vi "Load XCL template.vi"(9 "Template definition":T1={"Keywords column"=0, "Sig. freq. column"=1, "Rec. len. column"=2, "Meas. points. row min to read"=9, "Meas. points. row max to read"=1509, "Properties column"=4, "Properties row start"=1, "Properties row end"=5, "Keyword START regexp"="[Ss][Tt][Aa][Rr][Tt]", "Keyword STOP regexp"="[Ss][Tt][Oo][Pp]"}, 10 "Measurement template file":path, 11 "Measurement properties":T2={"Measurement frequencies (Hz)"=[1000.0, 10000.0, 1000.0], "Sampling frequency (Hz)"=500000.0, "Signal amplitude (V)"=4.5, "AC-DC settle time (s)"=20.0, "Record length (multiples of period)"=[1000.0, 10000.0, 1000.0], "Measurement template file"=path "", "Row of START keyword"=0, "Row of STOP keyword"=0, "Calculate RMS from samples"=FALSE, "AC-DC warm up time (s)"=300.0, "Measurement template line"=[], "DC meter readings No."=10} {"Record length (multiples of period)" format="%#_3p"; "Sampling frequency (Hz)" format="%#_3p"; "Measurement frequencies (Hz)" format="%#_3p"}) -> (3 "Measurement properties out":T2={"Measurement frequencies (Hz)"=[1000.0, 10000.0, 1000.0], "Sampling frequency (Hz)"=500000.0, "Signal amplitude (V)"=4.5, "AC-DC settle time (s)"=20.0, "Record length (multiples of period)"=[1000.0, 10000.0, 1000.0], "Measurement template file"=path "", "Row of START keyword"=0, "Row of STOP keyword"=0, "Calculate RMS from samples"=FALSE, "AC-DC warm up time (s)"=300.0, "Measurement template line"=[], "DC meter readings No."=10} {"Record length (multiples of period)" format="%#_3p"; "Sampling frequency (Hz)" format="%#_3p"; "Measurement frequencies (Hz)" format="%#_3p"})   [LabVIEW 2020]
doc: "Reads values from measurement template in excell spreadsheet."
uses:
  Measurement/Type definitions/Measuement properties.ctl
  Type definitions/Template definition.ctl
  <vilib>/Utility/NIReport.llb/Report Type.ctl
  <vilib>/Utility/error.llb/DialogType.ctl
  <vilib>/addons/_office/excel.llb/Excel Get Data ([str]).vi
  <vilib>/Utility/NIReport.llb/NI_report.lvclass
  <vilib>/addons/_office/NI_ReportGenerationToolkit.lvlib
  <vilib>/Utility/NIReport.llb/NI_ReportGenerationCore.lvlib
  <vilib>/Utility/NIReport.llb/Excel/NI_Excel.lvclass
panel:
  out "Stop row":i32
  out "Start row":i32
  out "excell template content":string[][](array[string])
  out "error out":errorcluster
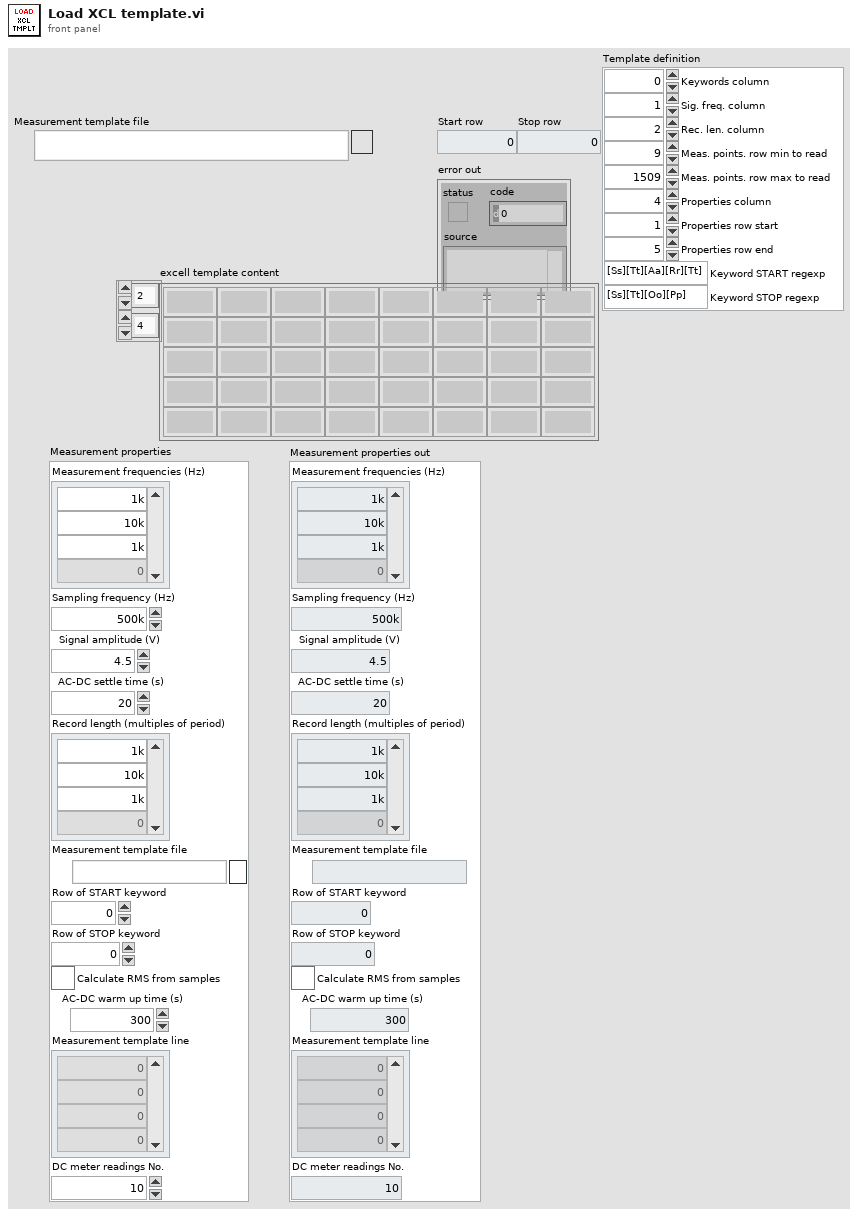
[diagram p1: front panel]
types:
  T1 = typedef "Template definition.ctl" = cluster{"Keywords column":i32, "Sig. freq. column":i32, "Rec. len. column":i32, "Meas. points. row min to read":i32, "Meas. points. row max to read":i32, "Properties column":i32, "Properties row start":i32, "Properties row end":i32, "Keyword START regexp":string, "Keyword STOP regexp":string}
  T2 = typedef "Measuement properties.ctl" = cluster{"Measurement frequencies (Hz)":dbl[], "Sampling frequency (Hz)":dbl, "Signal amplitude (V)":dbl, "AC-DC settle time (s)":dbl, "Record length (multiples of period)":dbl[], "Measurement template file":path, "Row of START keyword":i32, "Row of STOP keyword":i32, "Calculate RMS from samples":bool, "AC-DC warm up time (s)":dbl, "Measurement template line":i32[], "DC meter readings No.":i32}
  T3 = enum16{"maximized", "minimized", "normal", "no change"}
  T4 = typedef "NI_ReportGenerationCore.lvlib/Report Type.ctl" = enum16{"HTML", "Word", "Excel"}
  T5 = typedef "DialogType.ctl" = u16
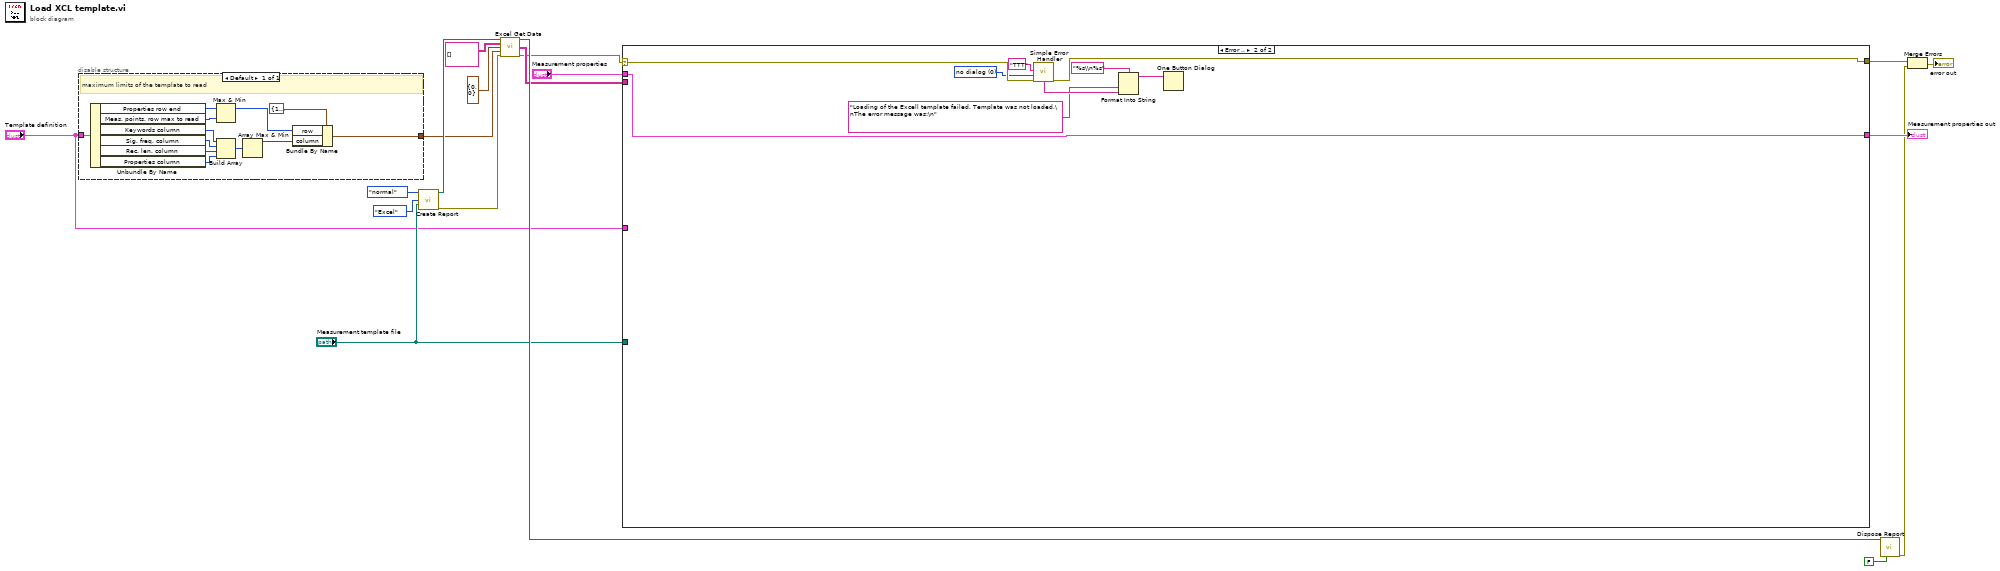
[diagram p0: block diagram]
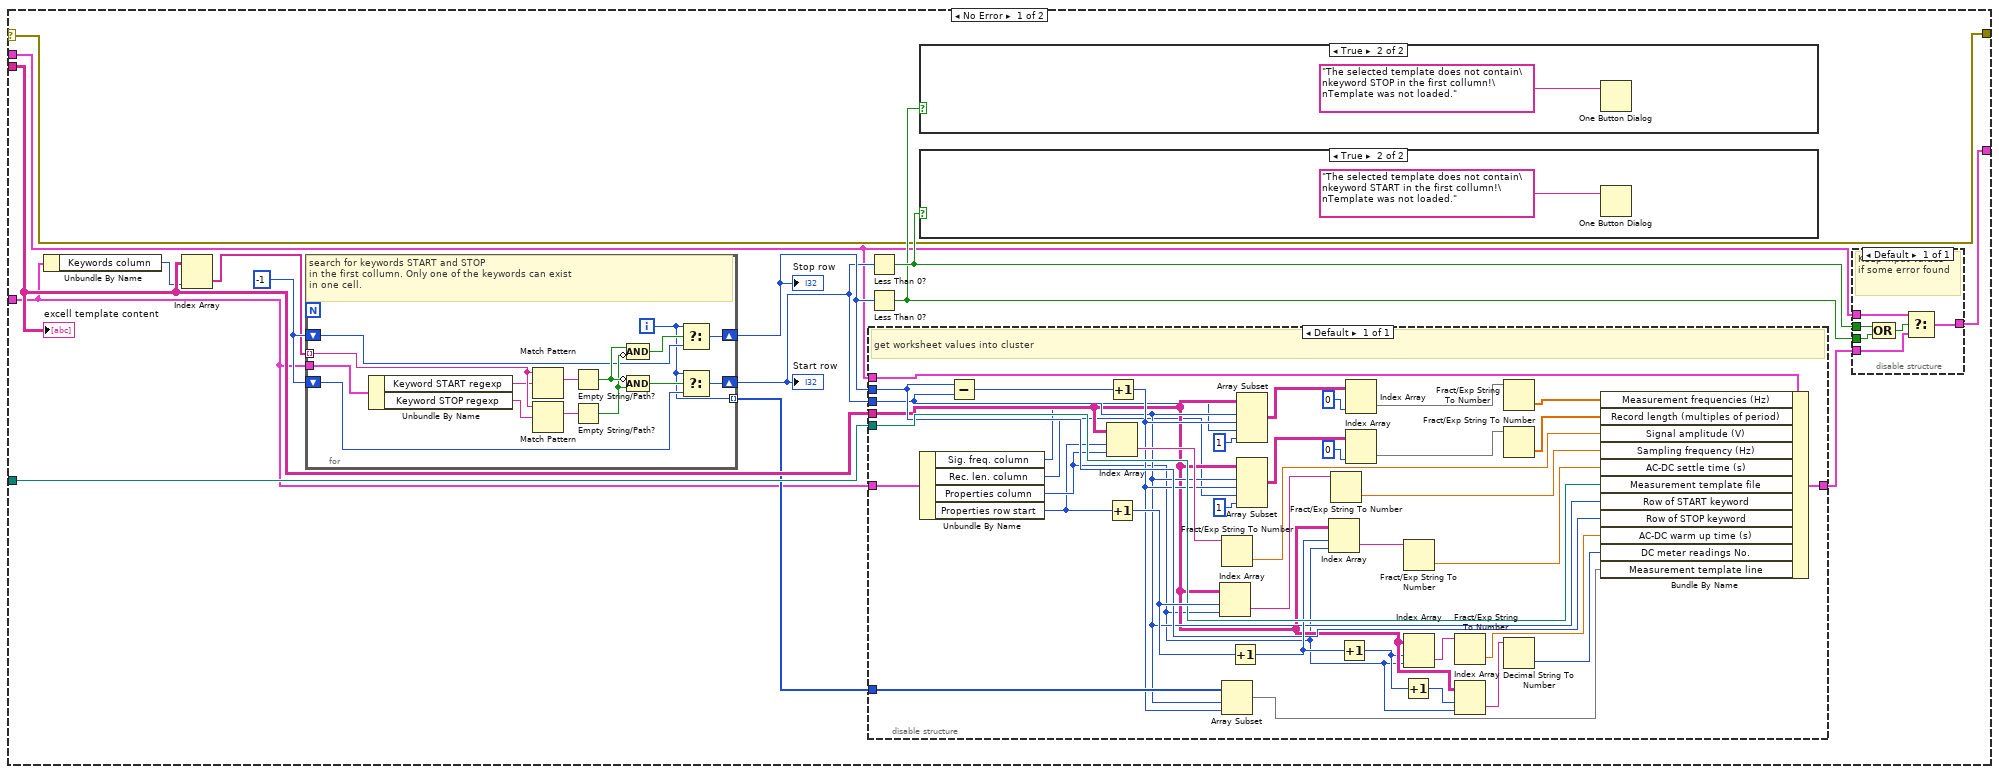
[diagram p2: hidden frame]
diagram:
  n1 = disable-structure shown="Default" {
    disable-tunnel: "Template definition" -> [w30]
    disable-tunnel: [w28] -> w2
    frame Enabled {
      # "maximum limits of the template to read"
      n2 = Unbundle By Name(w30) -> ("Properties row end"=w21:i32, "Meas. points. row max to read"=w20:i32, "Keywords column"=w27:i32, "Sig. freq. column"=w26:i32, "Rec. len. column"=w25:i32, "Properties column"=w24:i32)
      n3 = Max & Min(x=w21, y=w20) -> (max(x,y)=w19:i32)  [unwired: 1 out]
      n4 = Build Array(w27, w26, w25, w24) -> (w23:i32[])
      n5 = Array Max & Min(array=w23) -> (max value=w22:i32)  [unwired: 3 out]
      n6 = Bundle By Name(cluster=cluster{"row":i32, "column":i32} {"row"=100000, "column"=7} ("end (-1, -1)"), "row"=w19, "column"=w22) -> (w28:cluster{"row":i32, "column":i32})
    }
  }
  n7 = call <vilib>:"Create Report.vi"("window state (normal)"=T3."normal", "report type"=Report_Type."Excel", "template (empty)"="Measurement template file") -> ("report out"=w18:refnum<class "NI_report.lvclass">, "error out"=w17:errorcluster)  [unwired: 11 in]
  n8 = call-poly <vilib>:"Excel Get Data.vi"("report in"=w18, "data type"=string[][] [], "start (-1, -1)"=cluster{"row":i32, "column":i32} {"row"=0, "column"=0}, "end (-1, -1)"=w2, "error in (no error)"=w17) -> ("report out"=w16:refnum<class "NI_report.lvclass">, "data"=w12:string[][], "error out"=w6:errorcluster)  [unwired: 8 in]
  n9 = case shown="Error .." w6 {
    selector: w6 -> [w34 w115]
    tunnel: w12 -> [w41 _]
    tunnel: [w37 w116] -> w11
    tunnel: "Measurement properties" -> [w36 w116]
    tunnel: "Measurement template file" -> [w35 _]
    tunnel: [w34 w112] -> w5
    tunnel: "Template definition" -> [w32 _]
    frame No Error {
      w45 = -1
      n10 = Unbundle By Name(w32) -> ("Keywords column"=w31:i32)
      n11 = Index Array(array=w41, index (col)=w31) -> (element=w44:string[])  [unwired: 1 in]
      n12 = for {
        tunnel: w44 -> [w107] mode=indexing
        shift-right: [w103] -> w42
        shift-left: w45 -> [w97]
        shift-right: [w99] -> w43
        shift-left: w45 -> [w98]
        tunnel: [w96] -> w33 mode=indexing
        tunnel: w32 -> [w95]
        i -> [w96]
        # "search for keywords START and STOP\nin the first collumn. Only one of the keywords can exist\nin one cell."
        n13 = Unbundle By Name(w95) -> ("Keyword START regexp"=w94:string, "Keyword STOP regexp"=w93:string)
        n14 = Match Pattern(string=w107, regular expression=w94) -> (match substring=w106:string)  [unwired: 1 in, 3 out]
        n15 = Match Pattern(string=w107, regular expression=w93) -> (match substring=w105:string)  [unwired: 1 in, 3 out]
        n16 = Empty String/Path?(string/path=w106) -> (empty?=w102:bool)
        n17 = Empty String/Path?(string/path=w105) -> (empty?=w101:bool)
        n18 = Compound Arithmetic op=AND(w102, invert w101) -> (w100:bool)
        n19 = Compound Arithmetic op=AND(invert w102, w101) -> (w104:bool)
        n20 = Select(t=w96, s=w100, f=w98) -> (s? t:f=w99:i32)
        n21 = Select(t=w96, s=w104, f=w97) -> (s? t:f=w103:i32)
      }
      "Start row" <- w42
      "Stop row" <- w43
      n22 = Less Than 0?(x=w42) -> (x < 0?=w40:bool)
      n23 = Less Than 0?(x=w43) -> (x < 0?=w39:bool)
      n24 = disable-structure shown="Default" {
        disable-tunnel: w43 -> [w67]
        disable-tunnel: w42 -> [w63]
        disable-tunnel: w36 -> [w90]
        disable-tunnel: w41 -> [w59]
        disable-tunnel: [w84] -> w38
        disable-tunnel: w35 -> [w71]
        disable-tunnel: w33 -> [w66]
        disable-tunnel: w32 -> [w56]
        frame Enabled {
          # "get worksheet values into cluster"
          n25 = Unbundle By Name(w56) -> ("Sig. freq. column"=w55:i32, "Rec. len. column"=w54:i32, "Properties column"=w53:i32, "Properties row start"=w52:i32)
          n26 = Subtract(x=w67, y=w63) -> (x-y=w65:i32)
          n27 = Index Array(array=w59, index (row)=w52, index (col)=w53) -> (element=w78:string)
          n28 = Increment(x=w52) -> (x+1=w73:i32)
          n29 = Increment(x=w65) -> (x+1=w64:i32)
          n30 = Index Array(array=w59, index (row)=w73, index (col)=w53) -> (element=w76:string)
          n31 = Fract/Exp String To Number(string=w78) -> (number=w77:dbl)  [unwired: 3 in, 1 out]
          n32 = Array Subset(array=w66, index=w63, length=w64) -> (w62:i32[])
          n33 = Increment(x=w73) -> (x+1=w69:i32)
          n34 = Array Subset(array=w59, index (row)=w63, length (row)=w64, index (col)=w55, length (col)=1 ("length")) -> (w88:string[][])
          n35 = Array Subset(array=w59, index (row)=w63, length (row)=w64, index (col)=w54, length (col)=1 ("length")) -> (w81:string[][])
          n36 = Index Array(array=w59, index (row)=w69, index (col)=w53) -> (element=w74:string)
          n37 = Fract/Exp String To Number(string=w76) -> (number=w75:dbl)  [unwired: 3 in, 1 out]
          n38 = Increment(x=w69) -> (x+1=w58:i32)
          n39 = Index Array(array=w88, index (col)=0 ("index (row)")) -> (element=w86:string[])  [unwired: 1 in]
          n40 = Index Array(array=w81, index (col)=0 ("index (row)")) -> (element=w83:string[])  [unwired: 1 in]
          n41 = Increment(x=w58) -> (x+1=w61:i32)
          n42 = Fract/Exp String To Number(string=w74) -> (number=w72:dbl)  [unwired: 3 in, 1 out]
          n43 = Index Array(array=w59, index (row)=w58, index (col)=w53) -> (element=w70:string)
          n44 = Fract/Exp String To Number(string=w70) -> (number=w68:dbl)  [unwired: 3 in, 1 out]
          n45 = Index Array(array=w59, index (row)=w61, index (col)=w53) -> (element=w60:string)
          n46 = Fract/Exp String To Number(string=w86) -> (number=w85:dbl[])  [unwired: 3 in, 1 out]
          n47 = Fract/Exp String To Number(string=w83) -> (number=w79:dbl[])  [unwired: 3 in, 1 out]
          n48 = Decimal String To Number(string=w60) -> (number=w57:i32)  [unwired: 2 in, 1 out]
          n49 = Bundle By Name(cluster=w90, "Measurement frequencies (Hz)"=w85, "Record length (multiples of period)"=w79, "Signal amplitude (V)"=w77, "Sampling frequency (Hz)"=w75, "AC-DC settle time (s)"=w72, "Measurement template file"=w71, "Row of START keyword"=w63, "Row of STOP keyword"=w67, "AC-DC warm up time (s)"=w68, "DC meter readings No."=w57, "Measurement template line"=w62) -> (w84:T2)
        }
      }
      n50 = case shown="True" w39 {
        frame False {
        }
        frame True {
          n51 = One Button Dialog(message="The selected template does not contain\nkeyword STOP in the first collumn!\nTemplate was not loaded.") -> ()  [unwired: 1 in, 1 out]
        }
      }
      n52 = case shown="True" w40 {
        frame False {
        }
        frame True {
          n53 = One Button Dialog(message="The selected template does not contain\nkeyword START in the first collumn!\nTemplate was not loaded.") -> ()  [unwired: 1 in, 1 out]
        }
      }
      n54 = disable-structure shown="Default" {
        disable-tunnel: w40 -> [w50]
        disable-tunnel: w39 -> [w49]
        disable-tunnel: w38 -> [w48]
        disable-tunnel: [w47] -> w37
        disable-tunnel: w36 -> [w46]
        frame Enabled {
          # "Keep input values\nif some error found"
          n55 = Compound Arithmetic op=OR(w50, w49) -> (w51:bool)
          n56 = Select(t=w46, s=w51, f=w48) -> (s? t:f=w47:T2)
        }
      }
      "excell template content" <- w41
    }
    frame Error {
      w114 = T5 0 items=["no dialog", "OK message", "continue or stop message", "OK message + warnings", "continue/stop + warnings"] ("type of dialog (OK msg:1)")
      n57 = call <vilib>:"Simple Error Handler.vi"("error source (\" \")"="TTT" ("error source (\" \")"), "type of dialog (OK msg:1)"=w114, "error in (no error)"=w115) -> ("error out"=w112:errorcluster, "message"=w109:string)  [unwired: 2 in, 3 out]
      n58 = Format Into String(format string="%s\\n%s", "Loading of the Excell template failed. Template was not loaded.\nThe error message was:\n" ("input 1"), w109) -> (resulting string=w110:string)  [unwired: 2 in, 1 out]
      n59 = One Button Dialog(message=w110) -> ()  [unwired: 1 in, 1 out]
    }
  }
  "Measurement properties out" <- w11
  n60 = call-dynamic "Dispose Report.vi"("report in"=w16, "close report? (T)"=FALSE) -> ("error out"=w4:errorcluster)  [unwired: 13 in]
  n61 = Merge Errors(w5, w4) -> (→"error out":errorcluster)
